vi "freqToMs.vi"(11 "freq":dbl) -> (3 "ms":dbl)   [LabVIEW 2019]
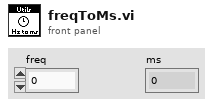
[diagram p1: front panel]
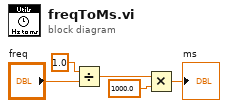
[diagram p0: block diagram]
diagram:
  n1 = Divide(x=1.0, y="freq") -> (x/y=w4:dbl)
  n2 = Multiply(x=w4, y=1000.0) -> (x*y=→"ms":dbl)
